vi "Assert Email.vi"() -> ()   [LabVIEW 2015, in "StmpEmail.lvclass"]
uses:
  StmpEmail.lvclass
panel:
  in  "Attachment Path":path=path "E:/LabVIEW相关/研究所培训计划/FirstDay/Demo1/src/Demo4/1. 视觉采集工具包的使用.vi"
  in  "Body:":string="asda"
  in  "Subject:":string="asd"
  in  "To: (email@site.com)":string="923371272@qq.com"
  in  "From: (email@site.com)":string="qianlingf@gmail.com"
  in  "Email Account Password":string="1110810220"
  in  "Email Account ID":string="qianlingf@gmail.com"
  in  "Port":i32=25
  in  "SMTP Outgoing Mail Server":string="smtp.gmail.com"
  in  "error in (no error)":errorcluster
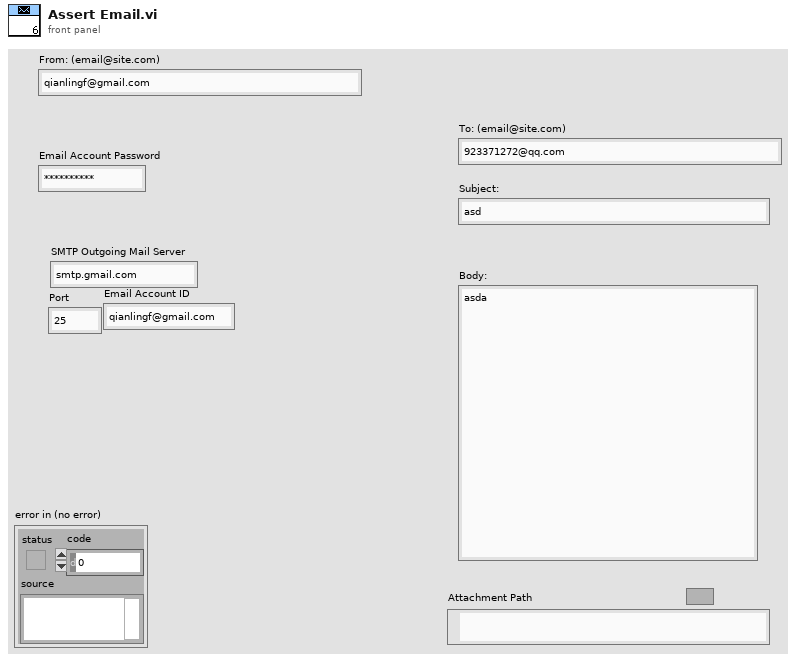
[diagram p1: front panel]
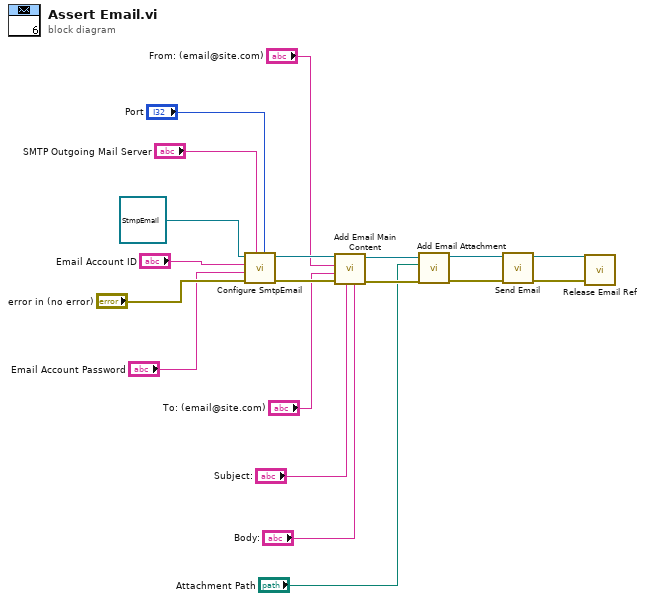
[diagram p0: block diagram]
diagram:
  n1 = call "Configure SmtpEmail.vi"("Port"="Port", "SMTP Outgoing Mail Server"="SMTP Outgoing Mail Server", "error in (no error)"="error in (no error)", "Email Account Password"="Email Account Password", "Email Account ID"="Email Account ID", "StmpEmail in"=refnum<class "StmpEmail.lvclass"> refnum ("StmpEmail.lvclass")) -> ("error out"=w17:errorcluster, "StmpEmail out"=w18:refnum<class "StmpEmail.lvclass">)  [unwired: 4 in]
  n2 = call "Add Email Main Content.vi"("Body:"="Body:", "Subject:"="Subject:", "error in (no error)"=w17, "To: (email@site.com)"="To: (email@site.com)", "From: (email@site.com)"="From: (email@site.com)", "StmpEmail in"=w18) -> ("error out"=w15:errorcluster, "StmpEmail out"=w16:refnum<class "StmpEmail.lvclass">)  [unwired: 4 in]
  n3 = call "Add Email Attachment.vi"("error in (no error)"=w15, "Attachment Path"="Attachment Path", "StmpEmail in"=w16) -> ("error out"=w13:errorcluster, "StmpEmail out"=w14:refnum<class "StmpEmail.lvclass">)  [unwired: 7 in]
  n4 = call "Send Email.vi"("error in (no error)"=w13, "StmpEmail in"=w14) -> ("error out"=w11:errorcluster, "StmpEmail out"=w12:refnum<class "StmpEmail.lvclass">)  [unwired: 8 in]
  n5 = call "Release Email Ref.vi"("error in (no error)"=w11, "StmpEmail in"=w12) -> ()  [unwired: 8 in, 2 out]
